vi "Send Message.vi"(8 "Error In":errorcluster caption="Fehler (Eingang)", 10 "Nachricht":string, 11 "Verbindungs-ID in":refnum<k16>) -> (0 "Error Out":errorcluster caption="Fehler (Ausgang)", 3 "Verbindungs-ID out":refnum<k16>)   [LabVIEW 2019, in "Thermostat Treiber.lvlib"]
uses:
  Thermostat Treiber.lvlib
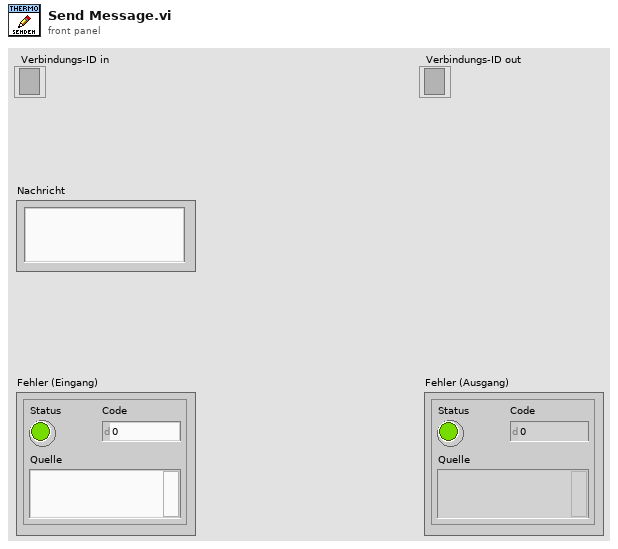
[diagram p1: front panel]
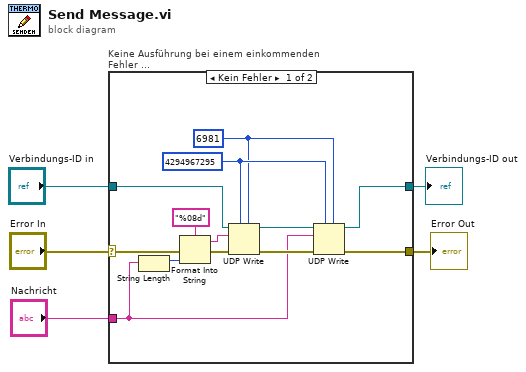
[diagram p0: block diagram]
diagram:
  n1 = case "Keine Ausführung bei einem einkommenden Fehler ..." shown="Kein Fehler" "Error In" {
    selector: "Error In" -> [w18 w20]
    tunnel: [w13 w20] -> w4
    tunnel: "Verbindungs-ID in" -> [w17 w19]
    tunnel: [w14 w19] -> w2
    tunnel: "Nachricht" -> [w10 _]
    frame No Error {
      w11 = u16 6981 ("Port oder Dienst")
      w12 = u32 4294967295 ("Adresse")
      n2 = String Length(string=w10) -> (length=w8:i32)
      n3 = Format Into String(format string="%08d" ("Format-String"), error in=w18, w8) -> (resulting string=w7:string, error out=w9:errorcluster)  [unwired: 1 in]
      n4 = UDP Write(address=w12, port or service name=w11, connection ID=w17, data in=w7, 8:w9) -> (error out=w16:errorcluster, 3:w15:refnum<k16>)  [unwired: 1 in]
      n5 = UDP Write(address=w12, port or service name=w11, connection ID=w15, data in=w10, 8:w16) -> (error out=w13:errorcluster, 3:w14:refnum<k16>)  [unwired: 1 in]
    }
    frame Error {
    }
  }
  "Error Out" <- w4
  "Verbindungs-ID out" <- w2
